vi "Write Path.vi"(5 "Path":path, 9 "SubVI in":refnum<class "SubVI.lvclass">) -> (3 "SubVI out":refnum<class "SubVI.lvclass">)   [LabVIEW 2014, in "Raspberry Pi Compatible Compiler for LabVIEW.lvlib" / "SubVI.lvclass"]
uses:
  SubVI.lvclass
  SubVI.lvclass/SubVI.ctl
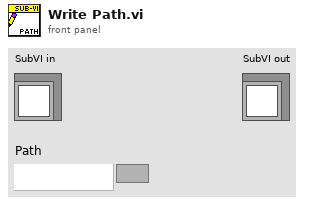
[diagram p1: front panel]
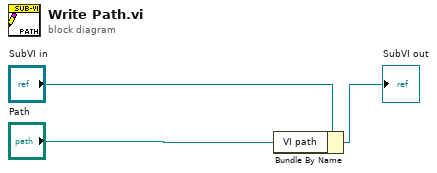
[diagram p0: block diagram]
diagram:
  n1 = Bundle By Name(cluster="SubVI in", "VI path"="Path") -> (→"SubVI out":refnum<class "SubVI.lvclass">)
